vi "Integrate 18bfxp1s.vi"(1 "G":fxp<+/-,18,1> format="%.18g") -> (0 "G/s":fxp<+/-,18,1> format="%.18g")   [LabVIEW 2009]
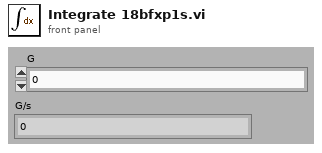
[diagram p1: front panel]
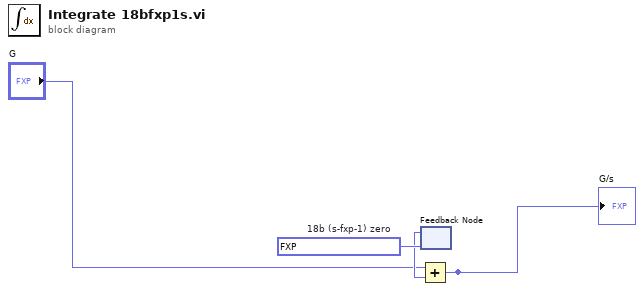
[diagram p0: block diagram]
diagram:
  w4 = fxp<+/-,18,1> 0.0  # 18b (s-fxp-1) zero
  n1 = feedback #1(w4) -> (w3:fxp<+/-,18,1>)
  n2 = Add ("Double Integrate Error")(x="G", y=w3) -> (x+y=w1:fxp<+/-,18,1>)
  "G/s" <- w1
